vi "QnFileName(SubVI).vi"() -> (0 "FileNames":string[](array[string]))   [LabVIEW 2013]
uses:
  FYP_LabviewGlobal(SubVI).vi
panel:
  out "Get Paper (-1 means not founded)":dbl
  out "Get Topic (-1 means not founded)":dbl
  out "Get Theme (-1 means not founded)":dbl
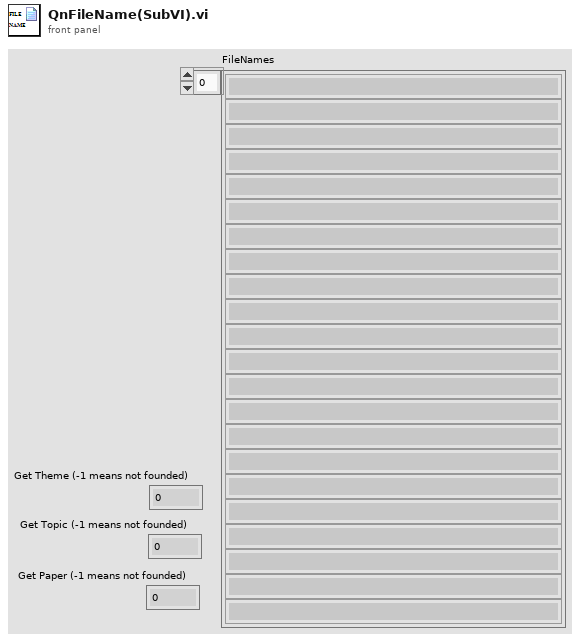
[diagram p1: front panel]
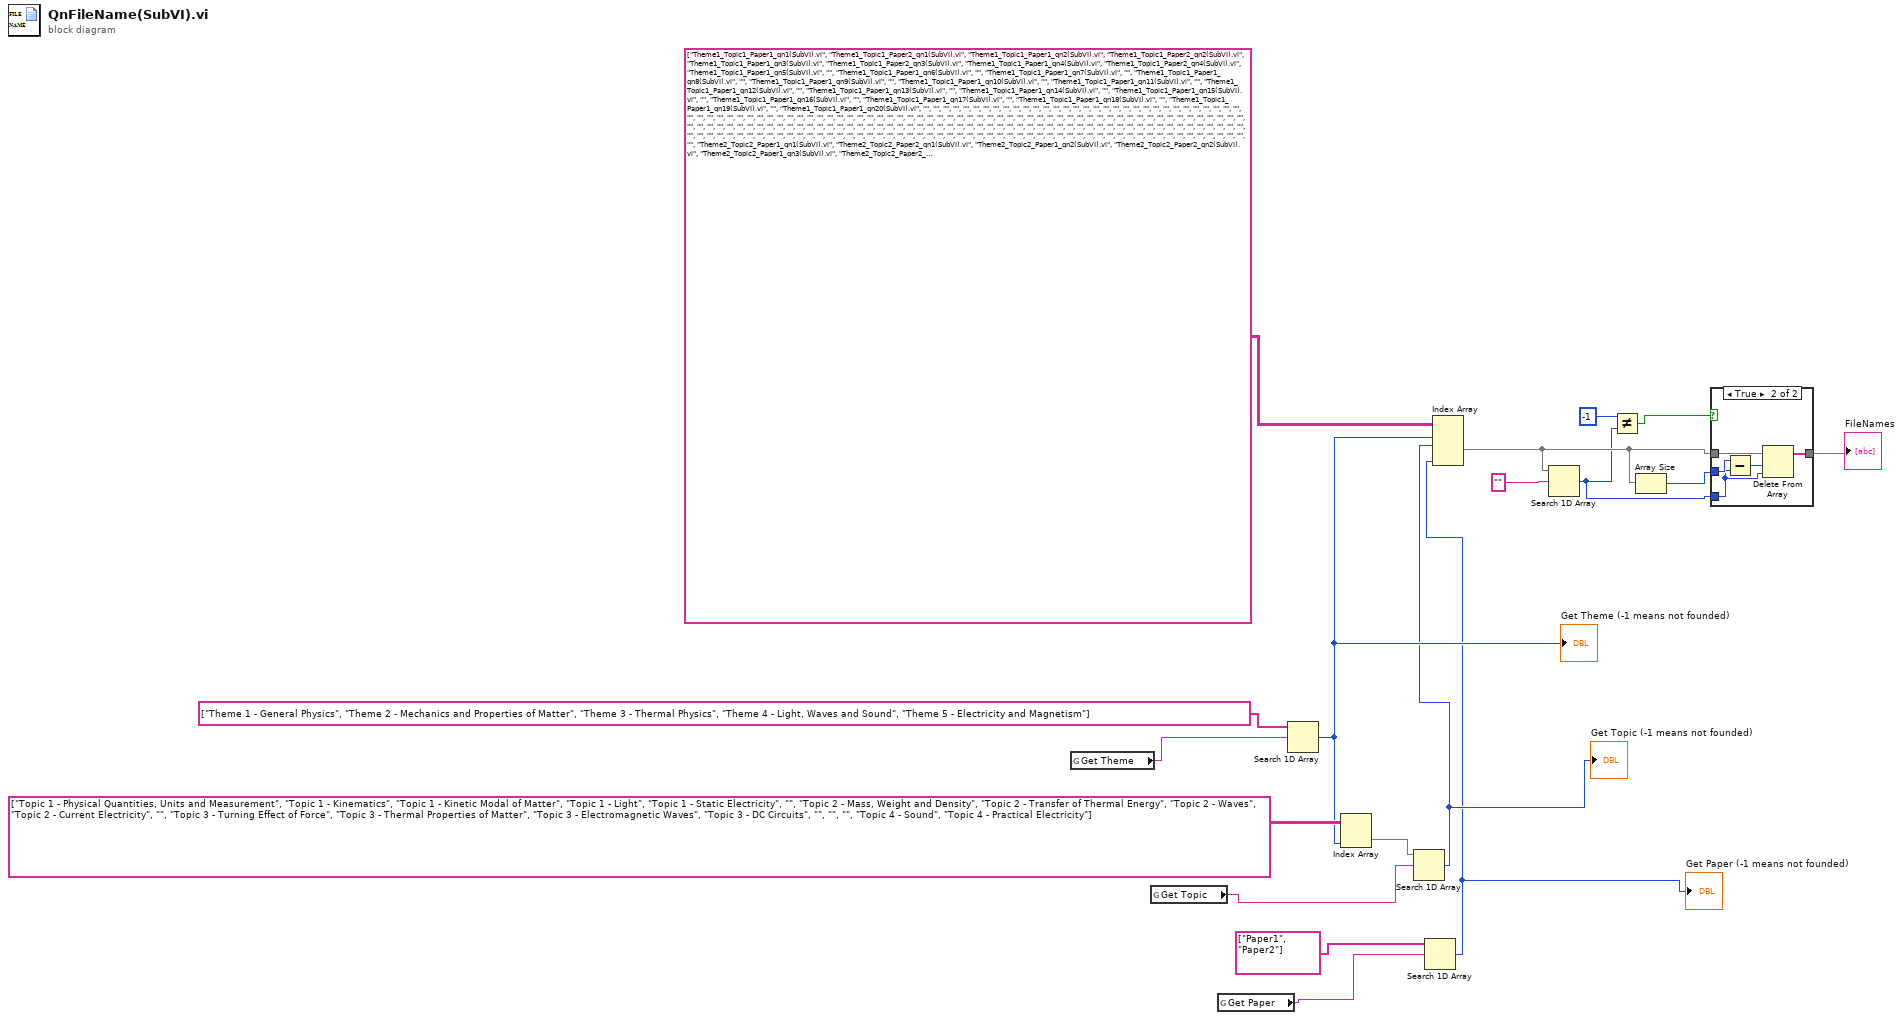
[diagram p0: block diagram]
diagram:
  n1 = global read "FYP_LabviewGlobal(SubVI).vi" "Get Theme"() -> (w3:string)
  n2 = global read "FYP_LabviewGlobal(SubVI).vi" "Get Topic"() -> (w2:string)
  n3 = global read "FYP_LabviewGlobal(SubVI).vi" "Get Paper"() -> (w1:string)
  n4 = Search 1D Array(1D array=string[] ["Theme 1 - General Physics", "Theme 2 - Mechanics and Properties of Matter", "Theme 3 - Thermal Physics", "Theme 4 - Light, Waves and Sound", "Theme 5 - Electricity and Magnetism"], element=w3) -> (index of element=w6:i32)  [unwired: 1 in]
  "Get Theme (-1 means not founded)" <- w6
  n5 = Index Array(array=string[][] [["Topic 1 - Physical Quantities, Units and Measurement", "Topic 1 - Kinematics", "Topic 1 - Kinetic Modal of Matter", "Topic 1 - Light", "Topic 1 - Static Electricity"], ["", "Topic 2 - Mass, Weight and Density", "Topic 2 - Transfer of Thermal Energy", "Topic 2 - Waves", "Topic 2 - Current Electricity"], ["", "Topic 3 - Turning Effect of Force", "Topic 3 - Thermal Properties of Matter", "Topic 3 - Electromagnetic Waves", "Topic 3 - DC Circuits"], ["", "", "", "Topic 4 - Sound", "Topic 4 - Practical Electricity"]], index (col)=w6) -> (element=w15:string[])  [unwired: 1 in]
  n6 = Search 1D Array(1D array=w15, element=w2) -> (index of element=w5:i32)  [unwired: 1 in]
  "Get Topic (-1 means not founded)" <- w5
  n7 = Search 1D Array(1D array=string[] ["Paper1", "Paper2"], element=w1) -> (index of element=w4:i32)  [unwired: 1 in]
  "Get Paper (-1 means not founded)" <- w4
  n8 = Index Array(array=string[][][][] [[[["Theme1_Topic1_Paper1_qn1(SubVI).vi", "Theme1_Topic1_Paper2_qn1(SubVI).vi"], ["Theme1_Topic1_Paper1_qn2(SubVI).vi", "Theme1_Topic1_Paper2_qn2(SubVI).vi"], ["Theme1_Topic1_Paper1_qn3(SubVI).vi", "Theme1_Topic1_Paper2_qn3(SubVI).vi"], ["Theme1_Topic1_Paper1_qn4(SubVI).vi", "Theme1_Topic1_Paper2_qn4(SubVI).vi"], ["Theme1_Topic1_Paper1_qn5(SubVI).vi", ""], ["Theme1_Topic1_Paper1_qn6(SubVI).vi", ""], ["Theme1_Topic1_Paper1_qn7(SubVI).vi", ""], ["Theme1_Topic1_Paper1_qn8(SubVI).vi", ""], ["Theme1_Topic1_Paper1_qn9(SubVI).vi", ""], ["Theme1_Topic1_Paper1_qn10(SubVI).vi", ""], ["Theme1_Topic1_Paper1_qn11(SubVI).vi", ""], ["Theme1_Topic1_Paper1_qn12(SubVI).vi", ""], ["Theme1_Topic1_Paper1_qn13(SubVI).vi", ""], ["Theme1_Topic1_Paper1_qn14(SubVI).vi", ""], ["Theme1_Topic1_Paper1_qn15(SubVI).vi", ""], ["Theme1_Topic1_Paper1_qn16(SubVI).vi", ""], ["Theme1_Topic1_Paper1_qn17(SubVI).vi", ""], ["Theme1_Topic1_Paper1_qn18(SubVI).vi", ""], ["Theme1_Topic1_Paper1_qn19(SubVI).vi", ""], ["Theme1_Topic1_Paper1_qn20(SubVI).vi", ""], ["", ""], ["", ""], ["", ""], ["", ""], ["", ""], ["", ""], ["", ""], ["", ""], ["", ""], ["", ""]], [["", ""], ["", ""], ["", ""], ["", ""], ["", ""], ["", ""], ["", ""], ["", ""], ["", ""], ["", ""], ["", ""], ["", ""], ["", ""], ["", ""], ["", ""], ["", ""], ["", ""], ["", ""], ["", ""], ["", ""], ["", ""], ["", ""], ["", ""], ["", ""], ["", ""], ["", ""], ["", ""], ["", ""], ["", ""], ["", ""]], [["", ""], ["", ""], ["", ""], ["", ""], ["", ""], ["", ""], ["", ""], ["", ""], ["", ""], ["", ""], ["", ""], ["", ""], ["", ""], ["", ""], ["", ""], ["", ""], ["", ""], ["", ""], ["", ""], ["", ""], ["", ""], ["", ""], ["", ""], ["", ""], ["", ""], ["", ""], ["", ""], ["", ""], ["", ""], ["", ""]], [["", ""], ["", ""], ["", ""], ["", ""], ["", ""], ["", ""], ["", ""], ["", ""], ["", ""], ["", ""], ["", ""], ["", ""], ["", ""], ["", ""], ["", ""], ["", ""], ["", ""], ["", ""], ["", ""], ["", ""], ["", ""], ["", ""], ["", ""], ["", ""], ["", ""], ["", ""], ["", ""], ["", ""], ["", ""], ["", ""]]], [[["Theme2_Topic2_Paper1_qn1(SubVI).vi", "Theme2_Topic2_Paper2_qn1(SubVI).vi"], ["Theme2_Topic2_Paper1_qn2(SubVI).vi", "Theme2_Topic2_Paper2_qn2(SubVI).vi"], ["Theme2_Topic2_Paper1_qn3(SubVI).vi", "Theme2_Topic2_Paper2_qn3(SubVI).vi"], ["Theme2_Topic2_Paper1_qn4(SubVI).vi", ""], ["Theme2_Topic2_Paper1_qn5(SubVI).vi", ""], ["Theme2_Topic2_Paper1_qn6(SubVI).vi", ""], ["Theme2_Topic2_Paper1_qn7(SubVI).vi", ""], ["Theme2_Topic2_Paper1_qn8(SubVI).vi", ""], ["Theme2_Topic2_Paper1_qn9(SubVI).vi", ""], ["Theme2_Topic2_Paper1_qn10(SubVI).vi", ""], ["Theme2_Topic2_Paper1_qn11(SubVI).vi", ""], ["Theme2_Topic2_Paper1_qn12(SubVI).vi", ""], ["Theme2_Topic2_Paper1_qn13(SubVI).vi", ""], ["Theme2_Topic2_Paper1_qn14(SubVI).vi", ""], ["Theme2_Topic2_Paper1_qn15(SubVI).vi", ""], ["", ""], ["", ""], ["", ""], ["", ""], ["", ""], ["", ""], ["", ""], ["", ""], ["", ""], ["", ""], ["", ""], ["", ""], ["", ""], ["", ""], ["", ""]], [["Theme2_Topic3_Paper1_qn1(SubVI).vi", "Theme2_Topic3_Paper2_qn1(SubVI).vi"], ["Theme2_Topic3_Paper1_qn2(SubVI).vi", "Theme2_Topic3_Paper2_qn2(SubVI).vi"], ["Theme2_Topic3_Paper1_qn3(SubVI).vi", "Theme2_Topic3_Paper2_qn3(SubVI).vi"], ["Theme2_Topic3_Paper1_qn4(SubVI).vi", "Theme2_Topic3_Paper2_qn4(SubVI).vi"], ["Theme2_Topic3_Paper1_qn5(SubVI).vi", ""], ["Theme2_Topic3_Paper1_qn6(SubVI).vi", ""], ["Theme2_Topic3_Paper1_qn7(SubVI).vi", ""], ["Theme2_Topic3_Paper1_qn8(SubVI).vi", ""], ["Theme2_Topic3_Paper1_qn9(SubVI).vi", ""], ["Theme2_Topic3_Paper1_qn10(SubVI).vi", ""], ["Theme2_Topic3_Paper1_qn11(SubVI).vi", ""], ["Theme2_Topic3_Paper1_qn12(SubVI).vi", ""], ["Theme2_Topic3_Paper1_qn13(SubVI).vi", ""], ["", ""], ["", ""], ["", ""], ["", ""], ["", ""], ["", ""], ["", ""], ["", ""], ["", ""], ["", ""], ["", ""], ["", ""], ["", ""], ["", ""], ["", ""], ["", ""], ["", ""]], [["Theme2_Topic4_Paper1_qn1(SubVI).vi", "Theme2_Topic4_Paper2_qn1(SubVI).vi"], ["", "Theme2_Topic4_Paper2_qn2(SubVI).vi"], ["", "Theme2_Topic4_Paper2_qn3(SubVI).vi"], ["", "Theme2_Topic4_Paper2_qn4(SubVI).vi"], ["", "Theme2_Topic4_Paper2_qn5(SubVI).vi"], ["", "Theme2_Topic4_Paper2_qn6(SubVI).vi"], ["", "Theme2_Topic4_Paper2_qn7(SubVI).vi"], ["", "Theme2_Topic4_Paper2_qn8(SubVI).vi"], ["", "Theme2_Topic4_Paper2_qn9(SubVI).vi"], ["", "Theme2_Topic4_Paper2_qn10(SubVI).vi"], ["", "Theme2_Topic4_Paper2_qn11(SubVI).vi"], ["", "Theme2_Topic4_Paper2_qn12(SubVI).vi"], ["", "Theme2_Topic4_Paper2_qn13(SubVI).vi"], ["", "Theme2_Topic4_Paper2_qn14(SubVI).vi"], ["", "Theme2_Topic4_Paper2_qn15(SubVI).vi"], ["", ""], ["", ""], ["", ""], ["", ""], ["", ""], ["", ""], ["", ""], ["", ""], ["", ""], ["", ""], ["", ""], ["", ""], ["", ""], ["", ""], ["", ""]], [["", ""], ["", ""], ["", ""], ["", ""], ["", ""], ["", ""], ["", ""], ["", ""], ["", ""], ["", ""], ["", ""], ["", ""], ["", ""], ["", ""], ["", ""], ["", ""], ["", ""], ["", ""], ["", ""], ["", ""], ["", ""], ["", ""], ["", ""], ["", ""], ["", ""], ["", ""], ["", ""], ["", ""], ["", ""], ["", ""]]], [[["Theme3_Topic1and2_qn1(SubVI).vi", ""], ["Theme3_Topic1and2_qn2(SubVI).vi", ""], ["Theme3_Topic1and2_qn3(SubVI).vi", ""], ["Theme3_Topic1and2_qn4(SubVI).vi", ""], ["Theme3_Topic1and2_qn5(SubVI).vi", ""], ["Theme3_Topic1and2_qn6(SubVI).vi", ""], ["Theme3_Topic1and2_qn7(SubVI).vi", ""], ["Theme3_Topic1and2_qn8(SubVI).vi", ""], ["Theme3_Topic1and2_qn9(SubVI).vi", ""], ["Theme3_Topic1and2_qn10(SubVI).vi", ""], ["Theme3_Topic1and2_qn11(SubVI).vi", ""], ["Theme3_Topic1and2_qn12(SubVI).vi", ""], ["Theme3_Topic1and2_qn13(SubVI).vi", ""], ["Theme3_Topic1and2_qn14(SubVI).vi", ""], ["Theme3_Topic1and2_qn15(SubVI).vi", ""], ["Theme3_Topic1and2_qn16(SubVI).vi", ""], ["Theme3_Topic1and2_qn17(SubVI).vi", ""], ["Theme3_Topic1and2_qn18(SubVI).vi", ""], ["Theme3_Topic1and2_qn19(SubVI).vi", ""], ["Theme3_Topic1and2_qn20(SubVI).vi", ""], ["Theme3_Topic1and2_qn21(SubVI).vi", ""], ["Theme3_Topic1and2_qn22(SubVI).vi", ""], ["Theme3_Topic1and2_qn23(SubVI).vi", ""], ["Theme3_Topic1and2_qn24(SubVI).vi", ""], ["Theme3_Topic1and2_qn25(SubVI).vi", ""], ["Theme3_Topic1and2_qn26(SubVI).vi", ""], ["Theme3_Topic1and2_qn27(SubVI).vi", ""], ["Theme3_Topic1and2_qn28(SubVI).vi", ""], ["Theme3_Topic1and2_qn29(SubVI).vi", ""], ["Theme3_Topic1and2_qn30(SubVI).vi", ""]], [["Theme3_Topic3_qn1(SubVI).vi", ""], ["Theme3_Topic3_qn2(SubVI).vi", ""], ["Theme3_Topic3_qn3(SubVI).vi", ""], ["Theme3_Topic3_qn4(SubVI).vi", ""], ["Theme3_Topic3_qn5(SubVI).vi", ""], ["Theme3_Topic3_qn6(SubVI).vi", ""], ["Theme3_Topic3_qn7(SubVI).vi", ""], ["Theme3_Topic3_qn8(SubVI).vi", ""], ["Theme3_Topic3_qn9(SubVI).vi", ""], ["Theme3_Topic3_qn10(SubVI).vi", ""], ["Theme3_Topic3_qn11(SubVI).vi", ""], ["Theme3_Topic3_qn12(SubVI).vi", ""], ["Theme3_Topic3_qn13(SubVI).vi", ""], ["Theme3_Topic3_qn14(SubVI).vi", ""], ["Theme3_Topic3_qn15(SubVI).vi", ""], ["Theme3_Topic3_qn16(SubVI).vi", ""], ["Theme3_Topic3_qn17(SubVI).vi", ""], ["Theme3_Topic3_qn18(SubVI).vi", ""], ["Theme3_Topic3_qn19(SubVI).vi", ""], ["Theme3_Topic3_qn20(SubVI).vi", ""], ["Theme3_Topic3_qn21(SubVI).vi", ""], ["Theme3_Topic3_qn22(SubVI).vi", ""], ["Theme3_Topic3_qn23(SubVI).vi", ""], ["Theme3_Topic3_qn24(SubVI).vi", ""], ["Theme3_Topic3_qn25(SubVI).vi", ""], ["Theme3_Topic3_qn26(SubVI).vi", ""], ["Theme3_Topic3_qn27(SubVI).vi", ""], ["Theme3_Topic3_qn28(SubVI).vi", ""], ["Theme3_Topic3_qn29(SubVI).vi", ""], ["Theme3_Topic3_qn30(SubVI).vi", ""]], [["Theme3_Topic4_qn1(SubVI).vi", "Theme3_Topic4_Paper2_qn1(SubVI).vi"], ["Theme3_Topic4_qn2(SubVI).vi", "Theme3_Topic4_Paper2_qn2(SubVI).vi"], ["Theme3_Topic4_qn3(SubVI).vi", "Theme3_Topic4_Paper2_qn3(SubVI).vi"], ["Theme3_Topic4_qn4(SubVI).vi", "Theme3_Topic4_Paper2_qn4(SubVI).vi"], ["Theme3_Topic4_qn5(SubVI).vi", "Theme3_Topic4_Paper2_qn5(SubVI).vi"], ["Theme3_Topic4_qn6(SubVI).vi", ""], ["Theme3_Topic4_qn7(SubVI).vi", ""], ["Theme3_Topic4_qn8(SubVI).vi", ""], ["Theme3_Topic4_qn9(SubVI).vi", ""], ["Theme3_Topic4_qn10(SubVI).vi", ""], ["Theme3_Topic4_qn11(SubVI).vi", ""], ["Theme3_Topic4_qn12(SubVI).vi", ""], ["Theme3_Topic4_qn13(SubVI).vi", ""], ["Theme3_Topic4_qn14(SubVI).vi", ""], ["Theme3_Topic4_qn15(SubVI).vi", ""], ["Theme3_Topic4_qn16(SubVI).vi", ""], ["Theme3_Topic4_qn17(SubVI).vi", ""], ["Theme3_Topic4_qn18(SubVI).vi", ""], ["Theme3_Topic4_qn19(SubVI).vi", ""], ["Theme3_Topic4_qn20(SubVI).vi", ""], ["Theme3_Topic4_qn21(SubVI).vi", ""], ["Theme3_Topic4_qn22(SubVI).vi", ""], ["Theme3_Topic4_qn23(SubVI).vi", ""], ["Theme3_Topic4_qn24(SubVI).vi", ""], ["Theme3_Topic4_qn25(SubVI).vi", ""], ["Theme3_Topic4_qn26(SubVI).vi", ""], ["Theme3_Topic4_qn27(SubVI).vi", ""], ["Theme3_Topic4_qn28(SubVI).vi", ""], ["Theme3_Topic4_qn29(SubVI).vi", ""], ["Theme3_Topic4_qn30(SubVI).vi", ""]], [["", ""], ["", ""], ["", ""], ["", ""], ["", ""], ["", ""], ["", ""], ["", ""], ["", ""], ["", ""], ["", ""], ["", ""], ["", ""], ["", ""], ["", ""], ["", ""], ["", ""], ["", ""], ["", ""], ["", ""], ["", ""], ["", ""], ["", ""], ["", ""], ["", ""], ["", ""], ["", ""], ["", ""], ["", ""], ["", ""]]], [[["Theme4_Topic1_qn1(SubVI).vi", ""], ["Theme4_Topic1_qn2(SubVI).vi", ""], ["Theme4_Topic1_qn3(SubVI).vi", ""], ["Theme4_Topic1_qn4(SubVI).vi", ""], ["Theme4_Topic1_qn5(SubVI).vi", ""], ["Theme4_Topic1_qn6(SubVI).vi", ""], ["Theme4_Topic1_qn7(SubVI).vi", ""], ["Theme4_Topic1_qn8(SubVI).vi", ""], ["Theme4_Topic1_qn9(SubVI).vi", ""], ["Theme4_Topic1_qn10(SubVI).vi", ""], ["Theme4_Topic1_qn11(SubVI).vi", ""], ["Theme4_Topic1_qn12(SubVI).vi", ""], ["Theme4_Topic1_qn13(SubVI).vi", ""], ["Theme4_Topic1_qn14(SubVI).vi", ""], ["Theme4_Topic1_qn15(SubVI).vi", ""], ["Theme4_Topic1_qn16(SubVI).vi", ""], ["Theme4_Topic1_qn17(SubVI).vi", ""], ["Theme4_Topic1_qn18(SubVI).vi", ""], ["Theme4_Topic1_qn19(SubVI).vi", ""], ["Theme4_Topic1_qn20(SubVI).vi", ""], ["Theme4_Topic1_qn21(SubVI).vi", ""], ["Theme4_Topic1_qn22(SubVI).vi", ""], ["Theme4_Topic1_qn23(SubVI).vi", ""], ["Theme4_Topic1_qn24(SubVI).vi", ""], ["Theme4_Topic1_qn25(SubVI).vi", ""], ["Theme4_Topic1_qn26(SubVI).vi", ""], ["Theme4_Topic1_qn27(SubVI).vi", ""], ["Theme4_Topic1_qn28(SubVI).vi", ""], ["Theme4_Topic1_qn29(SubVI).vi", ""], ["Theme4_Topic1_qn30(SubVI).vi", ""]], [["Theme4_Topic2_qn1(SubVI).vi", ""], ["Theme4_Topic2_qn2(SubVI).vi", ""], ["Theme4_Topic2_qn3(SubVI).vi", ""], ["Theme4_Topic2_qn4(SubVI).vi", ""], ["Theme4_Topic2_qn5(SubVI).vi", ""], ["Theme4_Topic2_qn6(SubVI).vi", ""], ["Theme4_Topic2_qn7(SubVI).vi", ""], ["Theme4_Topic2_qn8(SubVI).vi", ""], ["Theme4_Topic2_qn9(SubVI).vi", ""], ["Theme4_Topic2_qn10(SubVI).vi", ""], ["Theme4_Topic2_qn11(SubVI).vi", ""], ["Theme4_Topic2_qn12(SubVI).vi", ""], ["Theme4_Topic2_qn13(SubVI).vi", ""], ["Theme4_Topic2_qn14(SubVI).vi", ""], ["Theme4_Topic2_qn15(SubVI).vi", ""], ["Theme4_Topic2_qn16(SubVI).vi", ""], ["Theme4_Topic2_qn17(SubVI).vi", ""], ["Theme4_Topic2_qn18(SubVI).vi", ""], ["Theme4_Topic2_qn19(SubVI).vi", ""], ["Theme4_Topic2_qn20(SubVI).vi", ""], ["Theme4_Topic2_qn21(SubVI).vi", ""], ["Theme4_Topic2_qn22(SubVI).vi", ""], ["Theme4_Topic2_qn23(SubVI).vi", ""], ["Theme4_Topic2_qn24(SubVI).vi", ""], ["Theme4_Topic2_qn25(SubVI).vi", ""], ["Theme4_Topic2_qn26(SubVI).vi", ""], ["Theme4_Topic2_qn27(SubVI).vi", ""], ["Theme4_Topic2_qn28(SubVI).vi", ""], ["Theme4_Topic2_qn29(SubVI).vi", ""], ["Theme4_Topic2_qn30(SubVI).vi", ""]], [["Theme4_Topic3_qn1(SubVI).vi", ""], ["Theme4_Topic3_qn2(SubVI).vi", ""], ["Theme4_Topic3_qn3(SubVI).vi", ""], ["Theme4_Topic3_qn4(SubVI).vi", ""], ["Theme4_Topic3_qn5(SubVI).vi", ""], ["Theme4_Topic3_qn6(SubVI).vi", ""], ["Theme4_Topic3_qn7(SubVI).vi", ""], ["Theme4_Topic3_qn8(SubVI).vi", ""], ["Theme4_Topic3_qn9(SubVI).vi", ""], ["Theme4_Topic3_qn10(SubVI).vi", ""], ["Theme4_Topic3_qn11(SubVI).vi", ""], ["Theme4_Topic3_qn12(SubVI).vi", ""], ["Theme4_Topic3_qn13(SubVI).vi", ""], ["Theme4_Topic3_qn14(SubVI).vi", ""], ["Theme4_Topic3_qn15(SubVI).vi", ""], ["Theme4_Topic3_qn16(SubVI).vi", ""], ["Theme4_Topic3_qn17(SubVI).vi", ""], ["Theme4_Topic3_qn18(SubVI).vi", ""], ["Theme4_Topic3_qn19(SubVI).vi", ""], ["Theme4_Topic3_qn20(SubVI).vi", ""], ["Theme4_Topic3_qn21(SubVI).vi", ""], ["Theme4_Topic3_qn22(SubVI).vi", ""], ["Theme4_Topic3_qn23(SubVI).vi", ""], ["Theme4_Topic3_qn24(SubVI).vi", ""], ["Theme4_Topic3_qn25(SubVI).vi", ""], ["Theme4_Topic3_qn26(SubVI).vi", ""], ["Theme4_Topic3_qn27(SubVI).vi", ""], ["Theme4_Topic3_qn28(SubVI).vi", ""], ["Theme4_Topic3_qn29(SubVI).vi", ""], ["Theme4_Topic3_qn30(SubVI).vi", ""]], [["Theme4_Topic4_qn1(SubVI).vi", ""], ["Theme4_Topic4_qn2(SubVI).vi", ""], ["Theme4_Topic4_qn3(SubVI).vi", ""], ["Theme4_Topic4_qn4(SubVI).vi", ""], ["Theme4_Topic4_qn5(SubVI).vi", ""], ["Theme4_Topic4_qn6(SubVI).vi", ""], ["Theme4_Topic4_qn7(SubVI).vi", ""], ["Theme4_Topic4_qn8(SubVI).vi", ""], ["Theme4_Topic4_qn9(SubVI).vi", ""], ["Theme4_Topic4_qn10(SubVI).vi", ""], ["Theme4_Topic4_qn11(SubVI).vi", ""], ["Theme4_Topic4_qn12(SubVI).vi", ""], ["Theme4_Topic4_qn13(SubVI).vi", ""], ["Theme4_Topic4_qn14(SubVI).vi", ""], ["Theme4_Topic4_qn15(SubVI).vi", ""], ["Theme4_Topic4_qn16(SubVI).vi", ""], ["Theme4_Topic4_qn17(SubVI).vi", ""], ["Theme4_Topic4_qn18(SubVI).vi", ""], ["Theme4_Topic4_qn19(SubVI).vi", ""], ["Theme4_Topic4_qn20(SubVI).vi", ""], ["Theme4_Topic4_qn21(SubVI).vi", ""], ["Theme4_Topic4_qn22(SubVI).vi", ""], ["Theme4_Topic4_qn23(SubVI).vi", ""], ["Theme4_Topic4_qn24(SubVI).vi", ""], ["Theme4_Topic4_qn25(SubVI).vi", ""], ["Theme4_Topic4_qn26(SubVI).vi", ""], ["Theme4_Topic4_qn27(SubVI).vi", ""], ["Theme4_Topic4_qn28(SubVI).vi", ""], ["Theme4_Topic4_qn29(SubVI).vi", ""], ["Theme4_Topic4_qn30(SubVI).vi", ""]]], [[["Theme5_Topic1_qn1(SubVI).vi", ""], ["Theme5_Topic1_qn2(SubVI).vi", ""], ["Theme5_Topic1_qn3(SubVI).vi", ""], ["Theme5_Topic1_qn4(SubVI).vi", ""], ["Theme5_Topic1_qn5(SubVI).vi", ""], ["Theme5_Topic1_qn6(SubVI).vi", ""], ["Theme5_Topic1_qn7(SubVI).vi", ""], ["Theme5_Topic1_qn8(SubVI).vi", ""], ["Theme5_Topic1_qn9(SubVI).vi", ""], ["Theme5_Topic1_qn10(SubVI).vi", ""], ["Theme5_Topic1_qn11(SubVI).vi", ""], ["Theme5_Topic1_qn12(SubVI).vi", ""], ["Theme5_Topic1_qn13(SubVI).vi", ""], ["Theme5_Topic1_qn14(SubVI).vi", ""], ["Theme5_Topic1_qn15(SubVI).vi", ""], ["Theme5_Topic1_qn16(SubVI).vi", ""], ["Theme5_Topic1_qn17(SubVI).vi", ""], ["Theme5_Topic1_qn18(SubVI).vi", ""], ["Theme5_Topic1_qn19(SubVI).vi", ""], ["Theme5_Topic1_qn20(SubVI).vi", ""], ["Theme5_Topic1_qn21(SubVI).vi", ""], ["Theme5_Topic1_qn22(SubVI).vi", ""], ["Theme5_Topic1_qn23(SubVI).vi", ""], ["Theme5_Topic1_qn24(SubVI).vi", ""], ["Theme5_Topic1_qn25(SubVI).vi", ""], ["Theme5_Topic1_qn26(SubVI).vi", ""], ["Theme5_Topic1_qn27(SubVI).vi", ""], ["Theme5_Topic1_qn28(SubVI).vi", ""], ["Theme5_Topic1_qn29(SubVI).vi", ""], ["Theme5_Topic1_qn30(SubVI).vi", ""]], [["Theme5_Topic2_qn1(SubVI).vi", "Theme5_Topic2_Paper2_qn1(SubVI).vi"], ["Theme5_Topic2_qn2(SubVI).vi", "Theme5_Topic2_Paper2_qn2(SubVI).vi"], ["Theme5_Topic2_qn3(SubVI).vi", "Theme5_Topic2_Paper2_qn3(SubVI).vi"], ["Theme5_Topic2_qn4(SubVI).vi", ""], ["Theme5_Topic2_qn5(SubVI).vi", ""], ["Theme5_Topic2_qn6(SubVI).vi", ""], ["Theme5_Topic2_qn7(SubVI).vi", ""], ["Theme5_Topic2_qn8(SubVI).vi", ""], ["Theme5_Topic2_qn9(SubVI).vi", ""], ["Theme5_Topic2_qn10(SubVI).vi", ""], ["Theme5_Topic2_qn11(SubVI).vi", ""], ["Theme5_Topic2_qn12(SubVI).vi", ""], ["Theme5_Topic2_qn13(SubVI).vi", ""], ["Theme5_Topic2_qn14(SubVI).vi", ""], ["Theme5_Topic2_qn15(SubVI).vi", ""], ["Theme5_Topic2_qn16(SubVI).vi", ""], ["Theme5_Topic2_qn17(SubVI).vi", ""], ["Theme5_Topic2_qn18(SubVI).vi", ""], ["Theme5_Topic2_qn19(SubVI).vi", ""], ["Theme5_Topic2_qn20(SubVI).vi", ""], ["Theme5_Topic2_qn21(SubVI).vi", ""], ["Theme5_Topic2_qn22(SubVI).vi", ""], ["Theme5_Topic2_qn23(SubVI).vi", ""], ["Theme5_Topic2_qn24(SubVI).vi", ""], ["Theme5_Topic2_qn25(SubVI).vi", ""], ["Theme5_Topic2_qn26(SubVI).vi", ""], ["Theme5_Topic2_qn27(SubVI).vi", ""], ["Theme5_Topic2_qn28(SubVI).vi", ""], ["Theme5_Topic2_qn29(SubVI).vi", ""], ["Theme5_Topic2_qn30(SubVI).vi", ""]], [["Theme5_Topic3_qn1(SubVI).vi", "Theme5_Topic3_Paper2_qn1(SubVI).vi"], ["Theme5_Topic3_qn2(SubVI).vi", "Theme5_Topic3_Paper2_qn2(SubVI).vi"], ["Theme5_Topic3_qn3(SubVI).vi", "Theme5_Topic3_Paper2_qn3(SubVI).vi"], ["Theme5_Topic3_qn4(SubVI).vi", ""], ["Theme5_Topic3_qn5(SubVI).vi", ""], ["Theme5_Topic3_qn6(SubVI).vi", ""], ["Theme5_Topic3_qn7(SubVI).vi", ""], ["Theme5_Topic3_qn8(SubVI).vi", ""], ["Theme5_Topic3_qn9(SubVI).vi", ""], ["Theme5_Topic3_qn10(SubVI).vi", ""], ["Theme5_Topic3_qn11(SubVI).vi", ""], ["Theme5_Topic3_qn12(SubVI).vi", ""], ["Theme5_Topic3_qn13(SubVI).vi", ""], ["Theme5_Topic3_qn14(SubVI).vi", ""], ["Theme5_Topic3_qn15(SubVI).vi", ""], ["Theme5_Topic3_qn16(SubVI).vi", ""], ["Theme5_Topic3_qn17(SubVI).vi", ""], ["Theme5_Topic3_qn18(SubVI).vi", ""], ["Theme5_Topic3_qn19(SubVI).vi", ""], ["Theme5_Topic3_qn20(SubVI).vi", ""], ["Theme5_Topic3_qn21(SubVI).vi", ""], ["Theme5_Topic3_qn22(SubVI).vi", ""], ["Theme5_Topic3_qn23(SubVI).vi", ""], ["Theme5_Topic3_qn24(SubVI).vi", ""], ["Theme5_Topic3_qn25(SubVI).vi", ""], ["Theme5_Topic3_qn26(SubVI).vi", ""], ["Theme5_Topic3_qn27(SubVI).vi", ""], ["Theme5_Topic3_qn28(SubVI).vi", ""], ["Theme5_Topic3_qn29(SubVI).vi", ""], ["Theme5_Topic3_qn30(SubVI).vi", ""]], [["Theme5_Topic4_qn1(SubVI).vi", "Theme5_Topic4_Paper2_qn1(SubVI).vi"], ["Theme5_Topic4_qn2(SubVI).vi", "Theme5_Topic4_Paper2_qn2(SubVI).vi"], ["Theme5_Topic4_qn3(SubVI).vi", "Theme5_Topic4_Paper2_qn3(SubVI).vi"], ["Theme5_Topic4_qn4(SubVI).vi", ""], ["Theme5_Topic4_qn5(SubVI).vi", ""], ["Theme5_Topic4_qn6(SubVI).vi", ""], ["Theme5_Topic4_qn7(SubVI).vi", ""], ["Theme5_Topic4_qn8(SubVI).vi", ""], ["Theme5_Topic4_qn9(SubVI).vi", ""], ["Theme5_Topic4_qn10(SubVI).vi", ""], ["Theme5_Topic4_qn11(SubVI).vi", ""], ["Theme5_Topic4_qn12(SubVI).vi", ""], ["Theme5_Topic4_qn13(SubVI).vi", ""], ["Theme5_Topic4_qn14(SubVI)vi", ""], ["Theme5_Topic4_qn15(SubVI).vi", ""], ["Theme5_Topic4_qn16(SubVI).vi", ""], ["Theme5_Topic4_qn17(SubVI).vi", ""], ["Theme5_Topic4_qn18(SubVI).vi", ""], ["Theme5_Topic4_qn19(SubVI).vi", ""], ["Theme5_Topic4_qn20(SubVI).vi", ""], ["Theme5_Topic4_qn21(SubVI).vi", ""], ["Theme5_Topic4_qn22(SubVI).vi", ""], ["Theme5_Topic4_qn23(SubVI).vi", ""], ["Theme5_Topic4_qn24(SubVI).vi", ""], ["Theme5_Topic4_qn25(SubVI).vi", ""], ["Theme5_Topic4_qn26(SubVI).vi", ""], ["Theme5_Topic4_qn27(SubVI).vi", ""], ["Theme5_Topic4_qn28(SubVI).vi", ""], ["Theme5_Topic4_qn29(SubVI).vi", ""], ["Theme5_Topic4_qn30(SubVI).vi", ""]]]], index (dim 0)=w6, index (dim 1)=w5, index (dim 3)=w4) -> (element=w11:string[])  [unwired: 1 in]
  n9 = Search 1D Array(1D array=w11, element="") -> (index of element=w9:i32)  [unwired: 1 in]
  n10 = Not Equal?(x=-1 ("y"), y=w9) -> (x != y?=w8:bool)
  n11 = Array Size(array=w11) -> (size(s)=w10:i32)
  n12 = case shown="True" w8 {
    tunnel: w11 -> [w19 w24]
    tunnel: w10 -> [_ w23]
    tunnel: w9 -> [_ w22]
    tunnel: [w19 w20] -> w7
    frame False {
    }
    frame True {
      n13 = Subtract(x=w23, y=w22) -> (x-y=w21:i32)
      n14 = Delete From Array(array=w24, length=w21, index=w22) -> (array with subset deleted=w20:string[])  [unwired: 1 out]
    }
  }
  "FileNames" <- w7
